vi "Remove Termination.vi"(11 "String":string) -> (3 "substring":string)   [LabVIEW 2014, in "FIRST Events API.lvlib"]
uses:
  FIRST Events API.lvlib
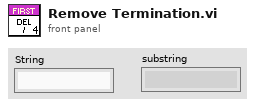
[diagram p1: front panel]
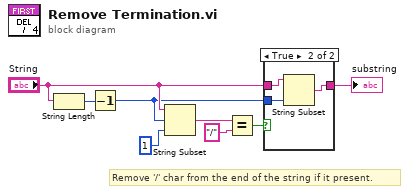
[diagram p0: block diagram]
diagram:
  # "Remove '/' char from the end of the string if it present."
  n1 = String Length(string="String") -> (length=w6:i32)
  n2 = Decrement(x=w6) -> (x-1=w2:i32)
  n3 = String Subset(string="String", offset (0)=w2, length (rest)=1 ("length (rest)")) -> (substring=w7:string)
  n4 = Equal?(x=w7, y="/") -> (x = y?=w5:bool)
  n5 = case shown="True" w5 {
    tunnel: "String" -> [w9 w12]
    tunnel: w2 -> [_ w11]
    tunnel: [w9 w10] -> w3
    frame False {
    }
    frame True {
      n6 = String Subset(string=w12, length (rest)=w11) -> (substring=w10:string)  [unwired: 1 in]
    }
  }
  "substring" <- w3
